vi "Read.vi"(8 "error in (no error)":errorcluster, 11 "VISA resource name":refnum<visa-resource-name>) -> (0 "error out":errorcluster, 1 "Current":dbl format="%_5g", 2 "Voltage":dbl format="%_6f", 3 "VISA resource name out":refnum<visa-resource-name>)   [LabVIEW 2024, in "BK Precision 8500B Series.lvlib"]
doc: "Reads back the measured voltage and current at the load input."
uses:
  BK Precision 8500B Series.lvlib
panel:
  # "V"
  # "A"
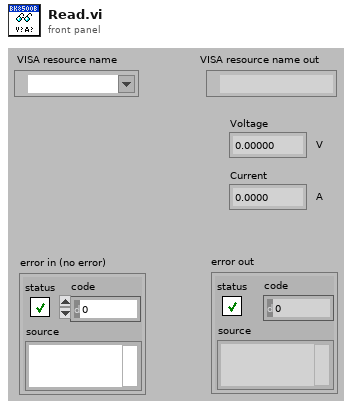
[diagram p1: front panel]
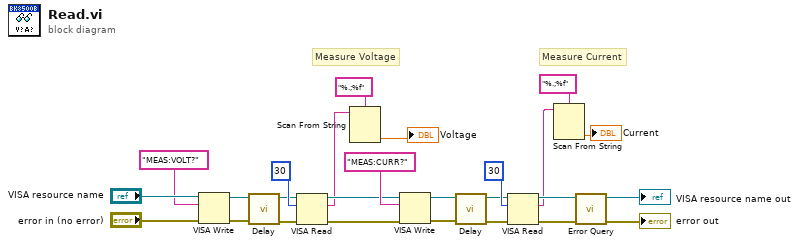
[diagram p0: block diagram]
diagram:
  # "Measure Current"
  # "Measure Voltage"
  n1 = VISA Write(VISA resource name="VISA resource name", write buffer="MEAS:VOLT?", error in (no error)="error in (no error)") -> (VISA resource name out=w8:refnum<visa-resource-name>, error out=w7:errorcluster)  [unwired: 1 out]
  n2 = call "Delay.vi"("error in (no error)"=w7, "VISA resource name"=w8) -> ("error out"=w10:errorcluster, "VISA resource name out"=w9:refnum<visa-resource-name>)  [unwired: 8 in]
  n3 = VISA Read(VISA resource name=w9, byte count=30, error in (no error)=w10) -> (VISA resource name out=w16:refnum<visa-resource-name>, read buffer=w14:string, error out=w15:errorcluster)  [unwired: 1 out]
  n4 = Scan From String(format string="%.;%f", input string=w14) -> (output 1=→"Voltage":dbl)  [unwired: 3 in, 3 out]
  n5 = VISA Write(VISA resource name=w16, write buffer="MEAS:CURR?", error in (no error)=w15) -> (VISA resource name out=w6:refnum<visa-resource-name>, error out=w5:errorcluster)  [unwired: 1 out]
  n6 = call "Delay.vi"("error in (no error)"=w5, "VISA resource name"=w6) -> ("error out"=w4:errorcluster, "VISA resource name out"=w3:refnum<visa-resource-name>)  [unwired: 8 in]
  n7 = VISA Read(VISA resource name=w3, byte count=30, error in (no error)=w4) -> (VISA resource name out=w24:refnum<visa-resource-name>, read buffer=w11:string, error out=w23:errorcluster)  [unwired: 1 out]
  n8 = Scan From String(format string="%.;%f", input string=w11) -> (output 1=→"Current":dbl)  [unwired: 3 in, 3 out]
  n9 = call "Error Query.vi"("error in (no error)"=w23, "VISA resource name"=w24) -> ("error out"=→"error out":errorcluster, "VISA resource name out"=→"VISA resource name out":refnum<visa-resource-name>)  [unwired: 6 in, 2 out]
